vi "lv_retrig-pulse-gen01-1.vi"() -> ()   [LabVIEW 2011]
doc: "I. Description:\nThis example demonstrates how to generate a finite digital pulse train from a Counter Output Channel. The Frequency, Duty Cycle, Initial Delay and Idle State are all configurable. This example uses two counters.\n\nThis example shows how to configure the pulse in terms of Frequency/Duty Cycle, but can easily be modified to generate a pulse in terms of Time or Ticks.\n\nII. Instructions for Running:\n1. Select the Physical Channel which corresponds to the counter you want to output your signal to on the DAQ device.\n2. Enter the Frequency and Duty Cycle to define the pulse parameters. Enter the Number Of Pulses into the DAQmx Timing VI to determine the duration of the generation (Note: if the Number of Pulses is greater than 1, the paired counter will also be used for the generation). Additionally, you can set the Initial Delay (in seconds) which will delay the beginning of the pulse train from the start call. Also, you can change the Idle State to set the state the line will remain in after the generation is stopped.\n3. Setup the Trigger Parameters. In this example the VI is expecting a Rising Edge Digital Trigger on PFI9 (ctr0 default gate).\nNote: Use the Measure Period example to verify you are outputting the finite pulse train on the DAQ device.\n \nIII. Block Diagram Steps:\n1. Create a Counter Output channel to produce a Pulse in terms of Frequency. If the Idle State of the pulse is set to low the first transition of the generated signal is from low to high.\n2. Use the DAQmx Timing VI (Implicit) to configure the duration of the pulse generation and the number of pulses to generate.\n3. Use the DAQmx Trigger VI to configure a trigger to start on a digital edge. \n4. Use a DAQmx Trigger Property Node to set the operation for retriggerable.\n5. Call the Start VI to arm the counter and begin the pulse train generation.\n6. Loop continuously until the user presses the Stop button. Check for errors every 100 ms using the Is Task Done? VI\n7. Call the Clear Task VI to clear the Task.\n8. Use the popup dialog box to display an error if any.\n\nIV. I/O Connections Overview:\nThe counter will output the pulse train on the output terminal of the counter specified in the Physical Channel I/O control. \n\nIn this example the output will be sent to the default output terminal on ctr0.\n\nFor more information on the default counter input and output terminals for your device, open the NI-DAQmx Help, and refer to Counter Signal Connections found under the Device Considerations book in the table of contents."
uses:
  <vilib>/Utility/error.llb/DialogType.ctl
  <vilib>/DAQmx/create/channels.llb/DAQmx Create Channel (CO-Pulse Generation-Frequency).vi
  <vilib>/DAQmx/configure/timing.llb/DAQmx Timing (Implicit).vi
  <vilib>/DAQmx/configure/trigger.llb/DAQmx Start Trigger (Digital Edge).vi
  Program Files/National Instruments/LabVIEW 2011/resource/objmgr/daqmx.rc
panel:
  in  "Stop":bool caption="stop"
  # "For instructions, select Help>>Show Context Help"
  # "Channel Parameters"
  # "Timing Parameters"
  # "Trigger Parameters"
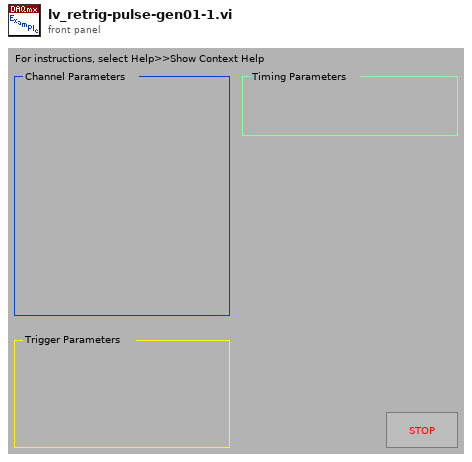
[diagram p1: front panel]
types:
  T1 = typedef "DialogType.ctl" = u16
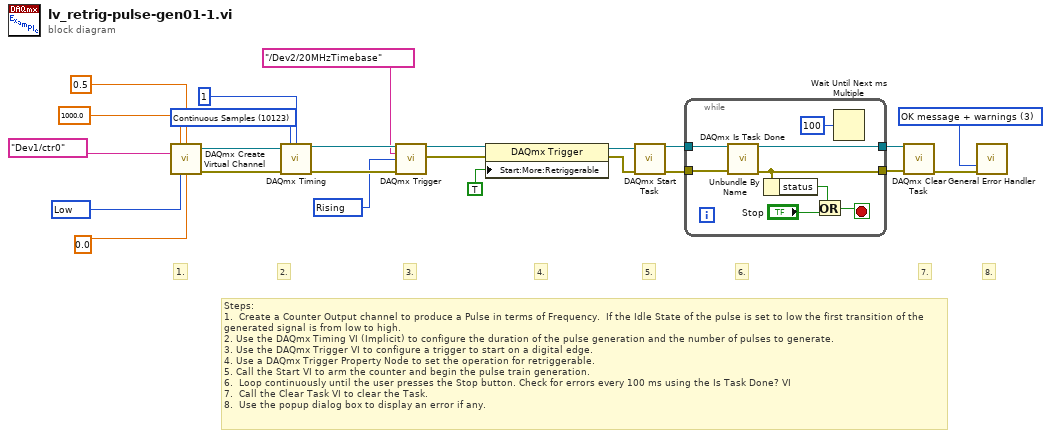
[diagram p0: block diagram]
diagram:
  w11 = 10280 items=["Rising"=10280, "Falling"=10171] ("Trigger Edge")
  w18 = 10214 items=["High"=10192, "Low"=10214] ("Idle State")
  w1 = T1 3 items=["no dialog", "OK message", "continue or stop message", "OK message + warnings", "continue/stop + warnings"] ("type of dialog (OK msg:1)")
  w21 = 10123 items=["Finite Samples"=10178, "Continuous Samples"=10123] ("sample mode")
  # "8."
  # "7."
  # "5."
  # "6."
  # "4."
  # "Steps: \n1.  Create a Counter Output channel to produce a Pulse in terms of Frequency.  If the Idle State of the pulse is set to low the first transition of the generated signal is from low to high.\n2. Use the DAQmx Timing VI (Implicit) to configure the duration of the pulse generation and the number of pulses to generate.\n3. Use the DAQmx Trigger VI to configure a trigger to start on a digital edge. \n4. Use a DAQmx Trigger Property Node to set the operation for retriggerable.\n5. Call the Start VI to arm the counter and begin the pulse train generation.\n6.  Loop continuously until the user presses the Stop button. Check for errors every 100 ms using the Is Task Done? VI\n7.  Call the Clear Task VI to clear the Task.\n8.  Use the popup dialog box to display an error if any."
  # "3."
  # "2."
  # "1."
  n1 = call-poly <vilib>:"DAQmx Create Virtual Channel.vi"("frequency"=1000.0 ("Frequency"), "duty cycle"=0.5 ("Duty Cycle"), "counter"=tag "Dev1/ctr0" ("Counter(s)"), "idle state"=w18, "initial delay"=0.0 ("Initial delay")) -> ("task out"=w22:refnum<k21>, "error out"=w24:errorcluster)  [unwired: 9 in]
  n2 = call-poly <vilib>:"DAQmx Timing.vi"("task/channels in"=w22, "sample mode"=w21, "samples per channel"=1 ("Number Of Pulses"), "error in"=w24) -> ("task out"=w14:refnum<k21>, "error out"=w13:errorcluster)  [unwired: 10 in]
  n3 = call-poly <vilib>:"DAQmx Trigger.vi"("task/channels in"=w14, "source"=tag "/Dev2/20MHzTimebase" ("Source"), "edge"=w11, "error in"=w13) -> ("task out"=w9:refnum<k21>, "error out"=w8:errorcluster)  [unwired: 10 in]
  n4 = property class="DAQmx Trigger"(reference=w9, error in=w8, "Start:More:Retriggerable"=TRUE) -> (reference out=w7:refnum<k21>, error out=w6:errorcluster)
  n5 = call <vilib>:"DAQmx Start Task.vi"("task/channels in"=w7, "error in"=w6) -> ("task out"=w5:refnum<k21>, "error out"=w4:errorcluster)  [unwired: 12 in]
  n6 = while {
    tunnel: [w25] -> w3
    tunnel: [w26] -> w2
    tunnel: w5 -> [w28]
    tunnel: w4 -> [w27]
    stop <- w30 stop-if-true
    n7 = call <vilib>:"DAQmx Is Task Done.vi"("task/channels in"=w28, "error in"=w27) -> ("task out"=w25:refnum<k21>, "error out"=w26:errorcluster)  [unwired: 11 in, 1 out]
    n8 = Unbundle By Name(w26) -> ("status"=w31:bool)
    n9 = Or(x=w31, y="Stop") -> (x .or. y?=w30:bool)
    n10 = Wait Until Next ms Multiple(millisecond multiple=u32 100) -> ()  [unwired: 1 out]
  }
  n11 = call <vilib>:"DAQmx Clear Task.vi"("task in"=w3, "error in"=w2) -> ("error out"=w23:errorcluster)  [unwired: 13 in]
  n12 = call <vilib>:"General Error Handler.vi"("type of dialog (OK msg:1)"=w1, "error in (no error)"=w23) -> ()  [unwired: 9 in, 5 out]
